vi "Подсчет числа вхождений алфавита.vi"(10 "Алфавит":string, 11 "Текст":string) -> (2 "Алфавит out":string, 3 "Число вхождений":i32[](array[numeric]))   [LabVIEW 2018]
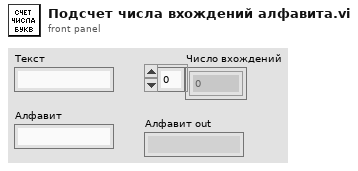
[diagram p1: front panel]
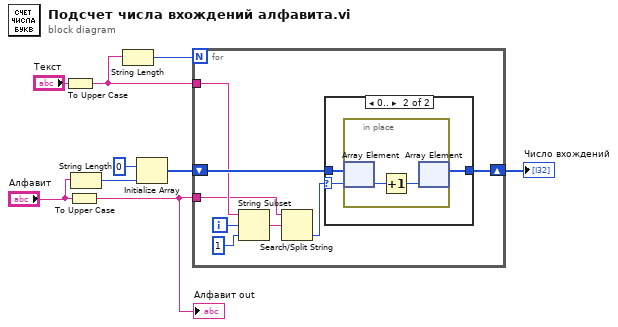
[diagram p0: block diagram]
diagram:
  n1 = To Upper Case(1:"Текст") -> (0:w6:string)
  n2 = To Upper Case(1:"Алфавит") -> (0:w8:string)
  "Алфавит out" <- w8
  n3 = String Length(string="Алфавит") -> (length=w3:i32)
  n4 = String Length(string=w6) -> (length=w5:i32)
  n5 = Initialize Array(0, w3) -> (w7:i32[])
  n6 = for {
    N: w5 -> [_]
    shift-right: [w16] -> w9
    shift-left: w7 -> [w17]
    tunnel: w6 -> [w15]
    tunnel: w8 -> [w12]
    i -> [w14]
    n7 = String Subset(string=w15, offset (0)=w14, length (rest)=1 ("length (rest)")) -> (substring=w11:string)
    n8 = Search/Split String(string=w12, search string/char (-)=w11) -> (offset of match=w10:i32)  [unwired: 1 in, 2 out]
    n9 = case shown="0.." w10 {
      selector: w10 -> [_ w20]
      tunnel: w17 -> [w18 w21]
      tunnel: [w18 w19] -> w16
      frame Default {
      }
      frame 0.. {
        n10 = in-place {
          n11 = in-place-array #1(w21, w20) -> (w23:i32)
          n12 = Increment(x=w23) -> (x+1=w22:i32)
          n13 = in-place-array #1(w22) -> (w19:i32[])  [unwired: 1 out]
        }
      }
    }
  }
  "Число вхождений" <- w9
